vi "sCAEN Read.vi"(0 "handle HV1":i32, 1 "handle HV2":i32, 2 "error in (no error)":errorcluster) -> (3 "handle HV1 out":i32, 4 "HV":sgl[](array[numeric]), 5 "handle HV2 out":i32, 6 "error out":errorcluster)   [LabVIEW 2014]
uses:
  CAEN/labview/CAENHVWrapper/CAENHVWrapper.lvlib
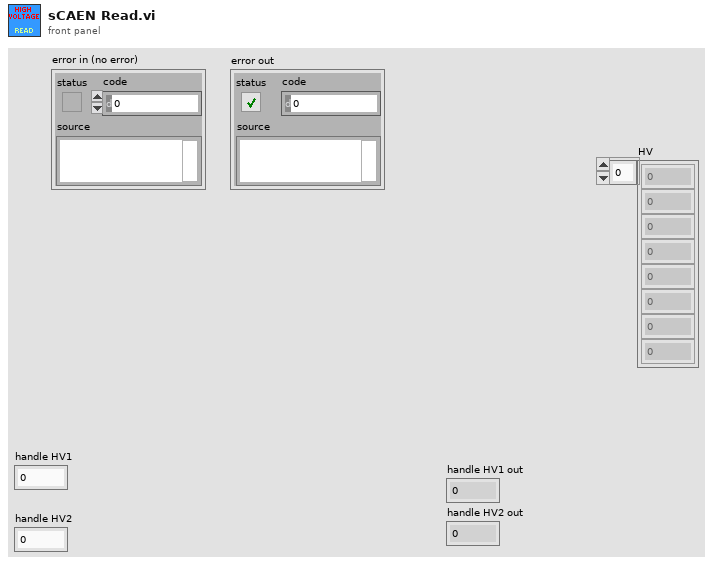
[diagram p1: front panel]
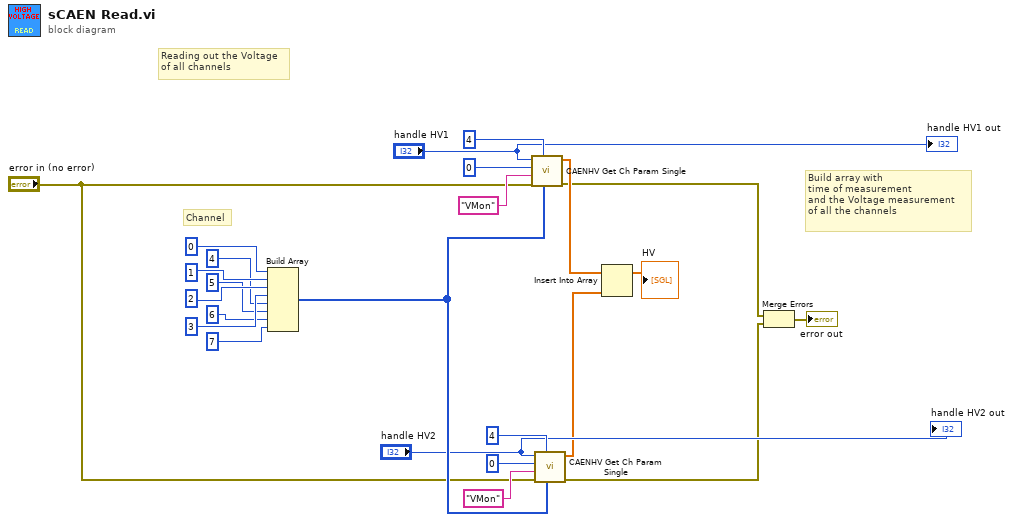
[diagram p0: block diagram]
diagram:
  # "Build array with \ntime of measurement \nand the Voltage measurement \nof all the channels"
  # "Channel"
  # "Reading out the Voltage\nof all channels"
  n1 = Build Array(0, 1, 2, 3, 4, 5, 6, 7) -> (w20:i32[])
  n2 = call "CAENHV Get Ch Param Single.vi"("ChList"=w20, "ChNum (1)"=u16 4, "error in (no error)"="error in (no error)", "ParName"="VMon", "slot"=u16 0, "handle"="handle HV1") -> ("error out"=w3:errorcluster, "ParValList"=w6:sgl[])  [unwired: 4 in]
  n3 = call "CAENHV Get Ch Param Single.vi"("ChList"=w20, "ChNum (1)"=u16 4, "error in (no error)"="error in (no error)", "ParName"="VMon", "slot"=u16 0, "handle"="handle HV2") -> ("error out"=w2:errorcluster, "ParValList"=w7:sgl[])  [unwired: 4 in]
  n4 = Insert Into Array(array=w6, new element=w7) -> (→"HV":sgl[])  [unwired: 1 in]
  n5 = Merge Errors(w3, w2) -> (→"error out":errorcluster)
  "handle HV1 out" <- "handle HV1"
  "handle HV2 out" <- "handle HV2"
